vi "Keithley 230 Coarse V ramp.vi"(5 "Time Interval (sec)":dbl=0.5 min=0.1 step=0.1, 6 "stop":bool, 7 "Sweep Time (H:M:S)":dbl=3600.0 format="%<%H:%M:%S>t", 8 "Mapping":bool, 9 "End Voltage (V)":dbl=1e-10 format="%.3e", 10 "Start Voltage (V)":dbl=1e-06 format="%.3e", 11 "Keithley 230 Address":refnum<visa-resource-name>) -> (1 "Last Sent Value":dbl=1e-06 format="%.3e")   [LabVIEW 2025]
doc: "Author: Scott Hannahs <sth@magnet.fsu.edu>\n\nThis software is licensed for use under the “MIT License\"\nCopyright (c) 2025 Scott Hannahs, sth@sth@magnet.sthnet.net\n\nPermission is hereby granted, free of charge, to any person obtaining a copy of this software and associated documentation files (the \"Software\"), to deal in the Software without restriction, including without limitation the rights to use, copy, modify, merge, publish, distribute, sublicense, and/or sell copies of the Software, and to permit persons to whom the Software is furnished to do so, subject to the following conditions: The above copyright notice and this permission notice shall be included in all copies or substantial portions of the Software.\n\nTHE SOFTWARE IS PROVIDED \"AS IS\", WITHOUT WARRANTY OF ANY KIND, EXPRESS OR IMPLIED, INCLUDING BUT NOT LIMITED TO THE WARRANTIES OF MERCHANTABILITY, FITNESS FOR A PARTICULAR PURPOSE AND NONINFRINGEMENT. IN NO EVENT SHALL THE AUTHORS OR COPYRIGHT HOLDERS BE LIABLE FOR ANY CLAIM, DAMAGES OR OTHER LIABILITY, WHETHER IN AN ACTION OF CONTRACT, TORT OR OTHERWISE, ARISING FROM, OUT OF OR IN CONNECTION WITH THE SOFTWARE OR THE USE OR OTHER DEALINGS IN THE SOFTWARE."
uses:
  Global Variables/Voltage K230 Coarse.vi
panel:
  out "Iteration":i32
  out "Prepared Value":dbl=1e-06 format="%.3e"
  # "Add two extra sec for timing."
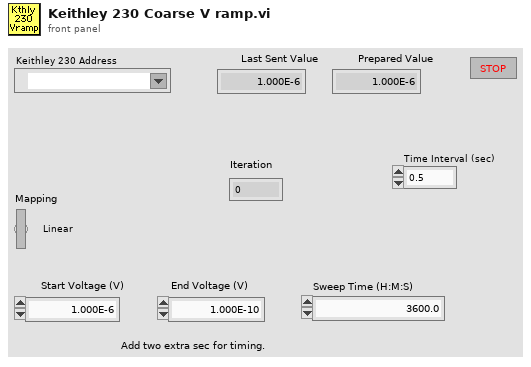
[diagram p1: front panel]
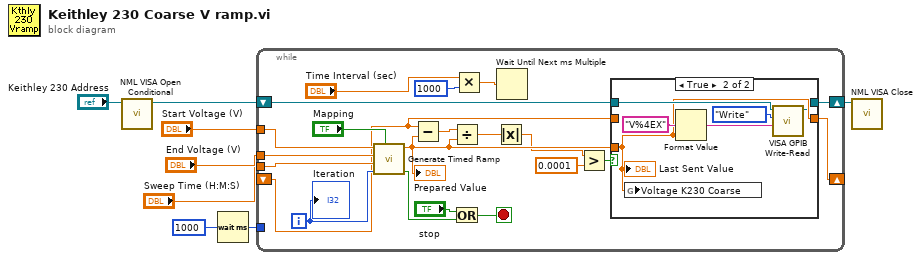
[diagram p0: block diagram]
diagram:
  n1 = call "NML VISA Open Conditional.vi"("VISA resource name"="Keithley 230 Address") -> ("dup VISA Session"=w3:refnum<visa-resource-name>)  [unwired: 8 in, 2 out]
  n2 = Wait (ms)(milliseconds to wait=u32 1000) -> (millisecond timer value=w2:u32)
  n3 = while {
    tunnel: "Start Voltage (V)" -> [w29]
    tunnel: "End Voltage (V)" -> [w28]
    tunnel: "Sweep Time (H:M:S)" -> [w27]
    shift-right: [w20] -> _
    shift-left: _ -> [w18]
    shift-right: [w9] -> w7
    shift-left: w3 -> [w16]
    tunnel: w2 -> [_]
    i -> [w26]
    stop <- w24 stop-if-true
    n4 = call "Generate Timed Ramp.vi"("Log"="Mapping", "Point #"=w26, "Time (Hr:Min:Sec)"=w27, "Stop"=w28, "Start"=w29) -> ("Stop"=w23:bool, "Output"=w17:dbl)  [unwired: 2 out]
    "Prepared Value" <- w17
    n5 = Subtract(x=w18, y=w17) -> (x-y=w12:dbl)
    n6 = Divide(x=w12, y=w17) -> (x/y=w11:dbl)
    n7 = Or(x="stop", y=w23) -> (x .or. y?=w24:bool)
    n8 = Multiply(x="Time Interval (sec)", y=u32 1000 ("millisecond multiple")) -> (x*y=w14:dbl)
    n9 = Absolute Value(x=w11) -> (abs(x)=w10:dbl)
    n10 = Wait Until Next ms Multiple(millisecond multiple=w14) -> ()  [unwired: 1 out]
    n11 = Greater?(x=w10, y=0.0001) -> (0:w19:bool)
    n12 = case shown="True" w19 {
      tunnel: [w31 w33] -> w20
      tunnel: w18 -> [w31 _]
      tunnel: w17 -> [_ w33]
      tunnel: w16 -> [w30 w34]
      tunnel: [w30 w32] -> w9
      frame False {
      }
      frame True {
        n13 = global write "Voltage K230 Coarse.vi" "Voltage K230 Coarse"(w33) -> ()
        n14 = Format Value(format string="V%4EX", value (0)=w33) -> (output string=w35:string)  [unwired: 1 in]
        n15 = call "VISA GPIB Write-Read.vi"("Command"=w35, "Action"=enum16{"Write", "Read", "Write & Read"}."Write", "VISA resource name"=w34) -> ("dup VISA Session"=w32:refnum<visa-resource-name>)  [unwired: 5 in, 3 out]
        "Last Sent Value" <- w33
      }
    }
    "Iteration" <- w26
  }
  n16 = call "NML VISA Close.vi"("VISA resource name"=w7) -> ()  [unwired: 10 in, 1 out]
